vi "EnemyKick2.vi"(6 "atacando contra?":bool, 8 "IA State Input 2":T1, 9 "balls":T4[](array[typedef]), 10 "Field Size in":T5, 11 "Robot in":T2) -> (3 "Robot out":T2)   [LabVIEW 2016]
uses:
  ROBOCUP/SSLVIEW/sslview/Core/Field Size.ctl
  ROBOCUP/SSLVIEW/sslview/Core/AI Robot.ctl
  ROBOCUP/SSLVIEW/sslview/Intel/Functions Enum.ctl
  ROBOCUP/SSLVIEW/sslview/Core/AI Ball.ctl
  ROBOCUP/SSLVIEW/sslview/Core/AI Input.ctl
  ROBOCUP/SSLVIEW/sslview/Core/AI Judge.ctl
  ROBOCUP/SSLVIEW/sslview/Intel/Command Enum.ctl
  <vilib>/Analysis/_algsub.llb/Real Vector Norm.vi
  <vilib>/Analysis/NI_AALPro.lvlib
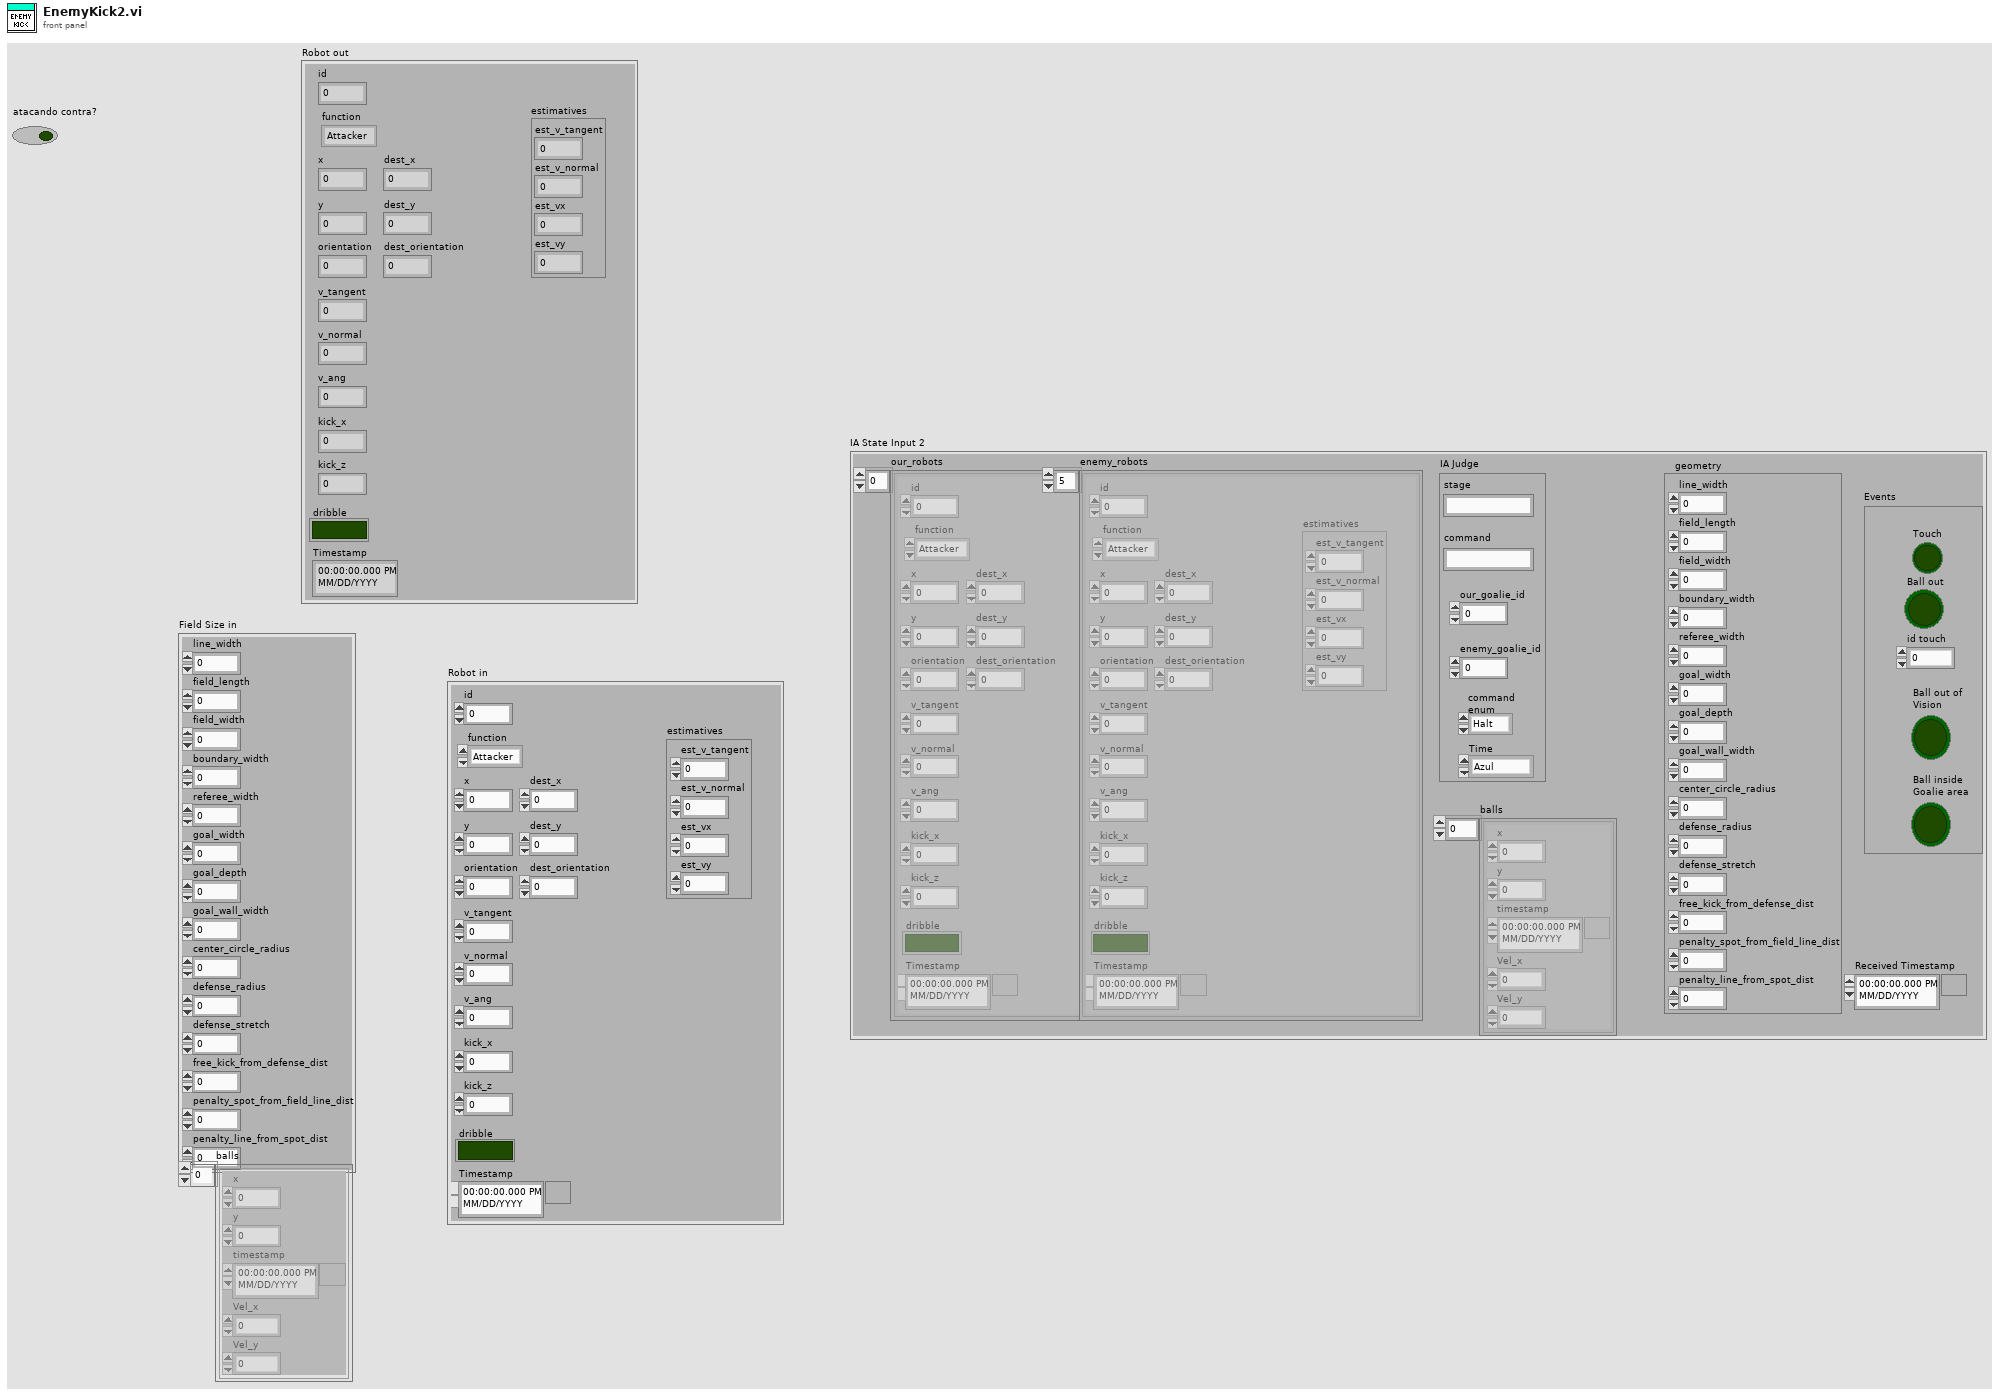
[diagram p1: front panel]
types:
  T1 = typedef "AI Input.ctl" = cluster{"our_robots":T2[], "enemy_robots":T2[], "balls":T4[], "geometry":T5, "IA Judge":T6, "Received Timestamp":timestamp, "Events":cluster{"Touch":bool, "Ball out":bool, "id touch":dbl, "Ball out of \nVision":bool, "Ball inside \nGoalie area":bool}}
  T2 = typedef "AI Robot.ctl" = cluster{"id":u32, "function":T3, "x":dbl, "y":dbl, "orientation":dbl, "v_tangent":dbl, "v_normal":dbl, "v_ang":dbl, "kick_x":dbl, "kick_z":dbl, "dribble":bool, "Timestamp":timestamp, "dest_x":dbl, "dest_y":dbl, "dest_orientation":dbl, "estimatives":cluster{"est_v_tangent":dbl, "est_v_normal":dbl, "est_vx":dbl, "est_vy":dbl}}
  T3 = typedef "Functions Enum.ctl" = enum16{"Attacker", "Goalie", "Defender", "Striker", "Goto 0", "Dummy", "ZigZag"}
  T4 = typedef "AI Ball.ctl" = cluster{"x":dbl, "y":dbl, "timestamp":timestamp, "Vel_x":dbl, "Vel_y":dbl}
  T5 = typedef "Field Size.ctl" = cluster{"line_width":u32, "field_length":u32, "field_width":u32, "boundary_width":u32, "referee_width":u32, "goal_width":u32, "goal_depth":u32, "goal_wall_width":u32, "center_circle_radius":u32, "defense_radius":u32, "defense_stretch":u32, "free_kick_from_defense_dist":u32, "penalty_spot_from_field_line_dist":u32, "penalty_line_from_spot_dist":u32}
  T6 = typedef "AI Judge.ctl" = cluster{"stage":string, "command":string, "our_goalie_id":dbl, "enemy_goalie_id":dbl, "command\nenum":T7, "Time":enum16{"Azul", "Amarelo"}}
  T7 = typedef "Command Enum.ctl" = enum16{"Halt", "Stop", "Force Start", "PKA Normal Start", "Prepare Kickoff Ally", "PKE Normal Start", "Prepare Kickoff Enemy", "Prepare Penalty Ally", "PPA Normal Start", "Prepare Penalty Enemy", "PPE Normal Start", "Direct Free Enemy", "Direct Free Ally", "Indirect Free Enemy", "Indirect Free Ally", "Timeout Enemy", "Timeout Ally", "Goal Enemy", "Goal Ally", "Ball Placement Enemy", "Ball Placement Ally", "None"}
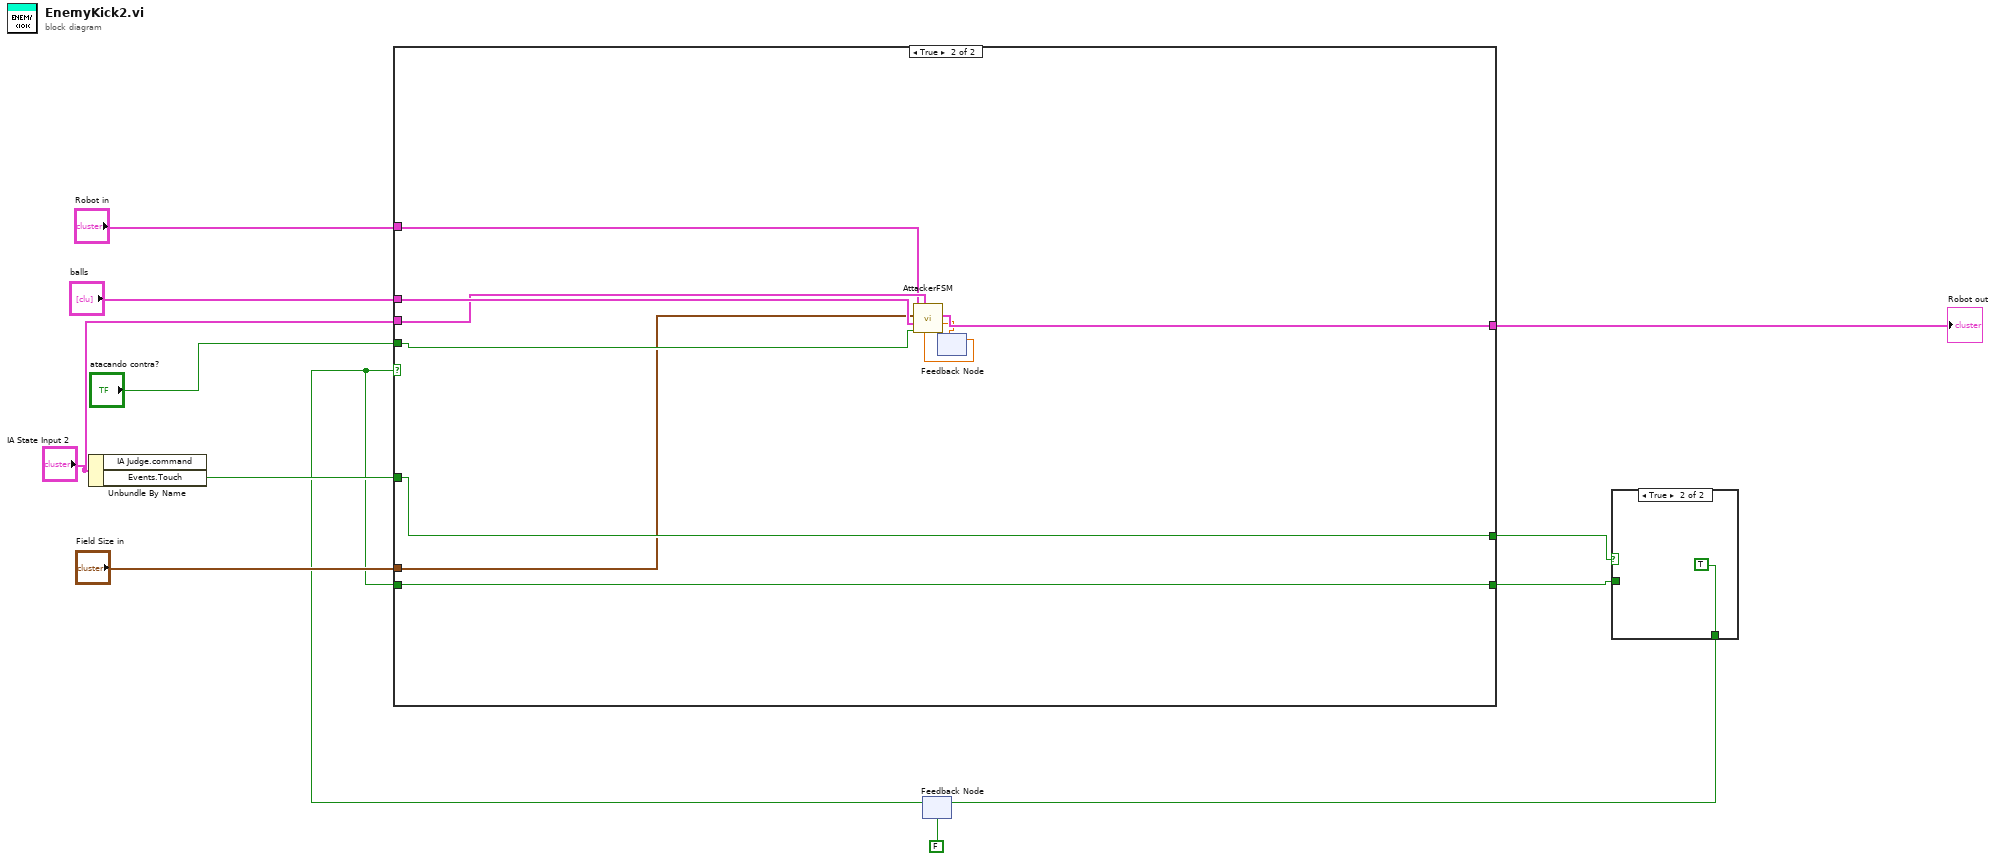
[diagram p0: block diagram]
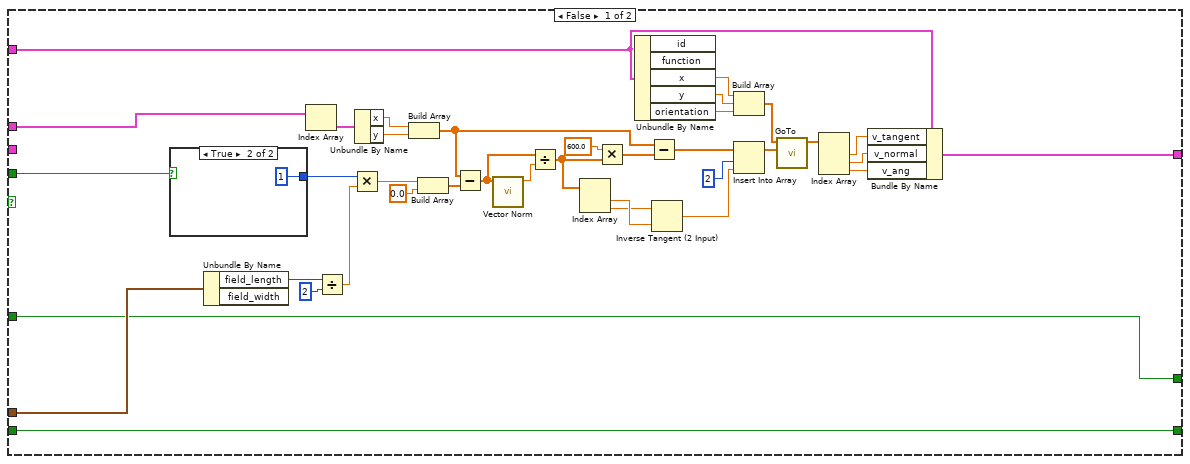
[diagram p3: hidden frame]
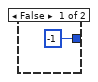
[diagram p4: hidden frame]
diagram:
  n1 = Unbundle By Name("IA State Input 2") -> ("Events.Touch"=w6:bool)  [unwired: 1 out]
  n2 = feedback #1(FALSE) -> (w2:bool)
  n3 = case shown="True" w2 {
    tunnel: "atacando contra?" -> [w41 w58]
    tunnel: [w36 w57] -> w11
    tunnel: "Robot in" -> [w35 w54]
    tunnel: "Field Size in" -> [w33 w55]
    tunnel: "balls" -> [w15 w59]
    tunnel: [w14 w61] -> w7
    tunnel: w6 -> [w14 w61]
    tunnel: [w13 w60] -> w3
    tunnel: w2 -> [w13 w60]
    tunnel: "IA State Input 2" -> [_ w56]
    frame False {
      n4 = case shown="True" w41 {
        tunnel: [-1 1] -> w29
        frame False {
        }
        frame True {
        }
      }
      n5 = Unbundle By Name(w33) -> ("field_length"=w49:u32)  [unwired: 1 out]
      n6 = Index Array(array=w15) -> (element=w45:T4)  [unwired: 1 in]
      n7 = Divide(x=w49, y=u32 2) -> (x/y=w40:dbl)
      n8 = Multiply(x=w29, y=w40) -> (x*y=w28:dbl)
      n9 = Unbundle By Name(w45) -> ("x"=w47:dbl, "y"=w46:dbl)
      n10 = Build Array(w47, w46) -> (w30:dbl[])
      n11 = Build Array(w28, 0.0 ("element")) -> (w24:dbl[])
      n12 = Subtract(x=w30, y=w24) -> (x-y=w25:dbl[])
      n13 = call-poly <vilib>:"Vector Norm.vi"("Input Vector"=w25) -> ("norm"=w26:dbl)  [unwired: 9 in, 1 out]
      n14 = Divide(x=w25, y=w26) -> (x/y=w19:dbl[])
      n15 = Index Array(array=w19) -> (element #1=w21:dbl, element #2=w20:dbl)  [unwired: 2 in]
      n16 = Multiply(x=600.0, y=w19) -> (x*y=w17:dbl[])
      n17 = Unbundle By Name(w35) -> ("x"=w44:dbl, "y"=w43:dbl, "orientation"=w42:dbl)  [unwired: 2 out]
      n18 = Subtract(x=w30, y=w17) -> (x-y=w16:dbl[])
      n19 = Inverse Tangent (2 Input)(1:w21, 2:w20) -> (0:w22:dbl)
      n20 = Build Array(w44, w43, w42) -> (w32:dbl[])
      n21 = Insert Into Array(array=w16, index=2, new element=w22) -> (w31:dbl[])
      n22 = call "GoTo.vi"("Target"=w31, "Position"=w32) -> ("Output\nVelocity"=w34:dbl[])  [unwired: 8 in, 1 out]
      n23 = Index Array(array=w34) -> (element #1=w37:dbl, element #2=w38:dbl, element #3=w39:dbl)  [unwired: 3 in]
      n24 = Bundle By Name(cluster=w35, "v_tangent"=w37, "v_normal"=w38, "v_ang"=w39) -> (w36:T2)
    }
    frame True {
      n25 = feedback #2() -> (w52:dbl)  [unwired: 1 in]
      n26 = call "AttackerFSM.vi"("Current State"=w52, "IA State Input 2"=w56, "atacando contra?"=w58, "balls"=w59, "Field Size in"=w55, "Robot in"=w54) -> ("Next State"=w53:dbl, "Robot out"=w57:T2)  [unwired: 4 in]
      n27 = feedback-in #2(w53) -> ()
    }
  }
  "Robot out" <- w11
  n28 = case shown="True" w7 {
    tunnel: [w62 TRUE] -> w5
    tunnel: w3 -> [w62 _]
    frame False {
    }
    frame True {
    }
  }
  n29 = feedback-in #1(w5) -> ()
